vi "实验2_4.vi"() -> ()   [LabVIEW 2018]
panel:
  in  "?":bool
  out "Success":cluster{"姓名":string, "学号":string}
  in  "Cluster":cluster{"姓名":string, " 学号":string, bool}={"姓名"="fcy", " 学号"="11111111", FALSE}
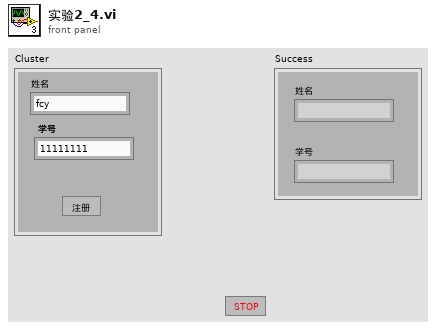
[diagram p1: front panel]
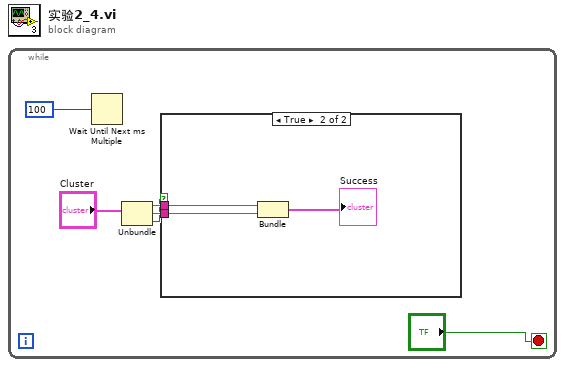
[diagram p0: block diagram]
diagram:
  n1 = while {
    stop <- "?" stop-if-true
    n2 = Wait Until Next ms Multiple(millisecond multiple=100) -> ()  [unwired: 1 out]
    n3 = Unbundle("Cluster") -> ("姓名"=w5:string, "学号"=w4:string, w3:bool)
    n4 = case shown="True" w3 {
      tunnel: w5 -> [_ w9]
      tunnel: w4 -> [_ w8]
      frame False {
      }
      frame True {
        n5 = Bundle("姓名"=w9, "学号"=w8) -> (→"Success":cluster{"姓名":string, " 学号":string})  [unwired: 1 in]
      }
    }
  }
